vi "getPollerPath.vi"(8 "error in (no error)":errorcluster, 11 "ttm_poller_panel.vi in":refnum<class "ttm_poller_panel.vi.lvclass">) -> (0 "error out":errorcluster, 2 "pollerPath":string, 3 "ttm_poller_panel.vi out":refnum<class "ttm_poller_panel.vi.lvclass">)   [LabVIEW 2009]
uses:
  ttm_poller_panel.vi.lvclass
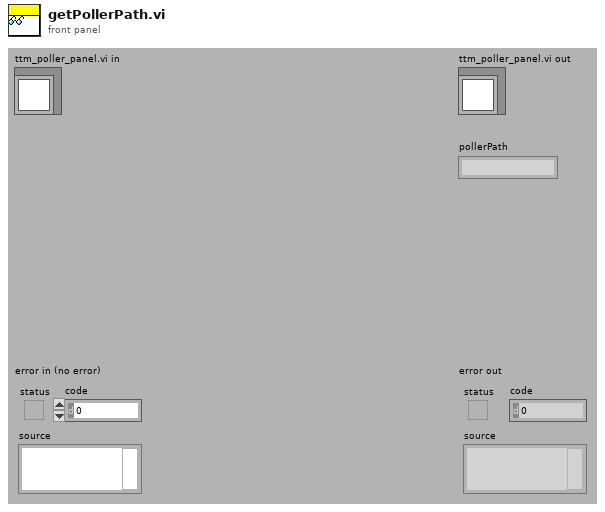
[diagram p1: front panel]
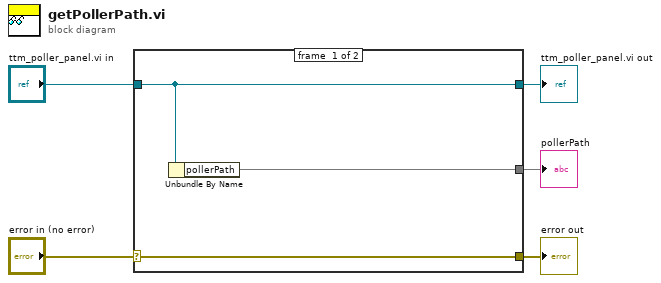
[diagram p0: block diagram]
diagram:
  n1 = case shown="No Error" "error in (no error)" {
    selector: "error in (no error)" -> [w8 w9]
    tunnel: [w8 w9] -> w4
    tunnel: [w7 w10] -> w2
    tunnel: "ttm_poller_panel.vi in" -> [w7 w10]
    tunnel: [w6 _] -> w1
    frame #0 {
      n2 = Unbundle By Name(w7) -> ("pollerPath"=w6)
    }
    frame #1 {
    }
  }
  "error out" <- w4
  "ttm_poller_panel.vi out" <- w2
  "pollerPath" <- w1
